vi "GetDriveQueue.vi"(8 "error in (no error)":errorcluster) -> (0 "error out":errorcluster, 3 "queue out":refnum<queue>)   [LabVIEW 2013]
uses:
  DriveQueueInstruction.ctl
  DriveInstruction.ctl
  QueueSubsystem.ctl
  KariFramework/TankDriveAction.ctl
panel:
  out "created new?":bool
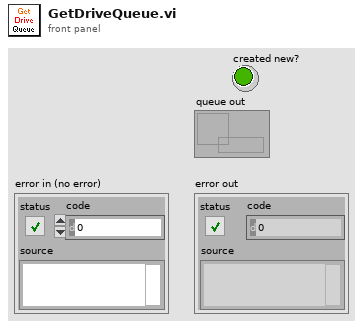
[diagram p1: front panel]
types:
  T1 = typedef "DriveQueueInstruction.ctl" = cluster{"DriveInstruction":T2, "Subsystem":T3, "Action":T4, "LoopTiming":u32}
  T2 = typedef "DriveInstruction.ctl" = cluster{"cDriveLeft":dbl, "cDriveRight":dbl, "cHalfDrive":bool, "cStraightDrive":bool}
  T3 = typedef "QueueSubsystem.ctl" = enum16{"Drive", "Arm", "Catapult", "Roller"}
  T4 = typedef "TankDriveAction.ctl" = enum16{"Init", "LinearDrive", "SetValue", "Disable"}
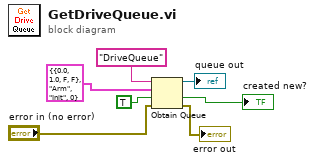
[diagram p0: block diagram]
diagram:
  n1 = Obtain Queue(name (unnamed)="DriveQueue", element data type=T1 {"DriveInstruction"={"cDriveLeft"=0.0, "cDriveRight"=1.0, "cHalfDrive"=FALSE, "cStraightDrive"=FALSE}, "Subsystem"=enum."Arm", "Action"=enum."Init", "LoopTiming"=0} ("Cluster"), create if not found? (T)=TRUE, error in (no error)="error in (no error)") -> (queue out=→"queue out":refnum<queue>, created new?=→"created new?":bool, error out=→"error out":errorcluster)  [unwired: 1 in]
